vi "CRYReport Pic Get License.vi"() -> (0 "363d8b37-68c8-11db-be1e-0013d350667c":string, 2 "363d8b35-68c8-11db-be1e-0013d350667c":string)   [LabVIEW 2013]
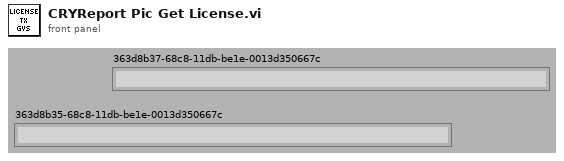
[diagram p1: front panel]
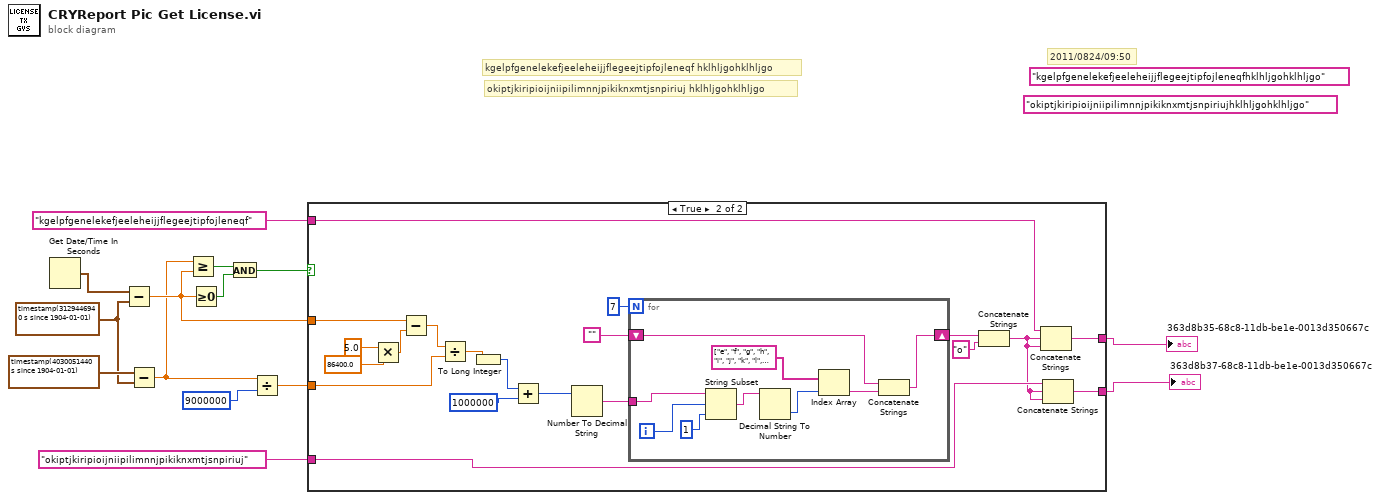
[diagram p0: block diagram]
diagram:
  w6 = timestamp(3129446940 s since 1904-01-01) ("current time")
  (unwired) "okiptjkiripioijniipilimnnjpikiknxmtjsnpiriujhklhljgohklhljgo"
  (unwired) "kgelpfgenelekefjeeleheijjflegeejtipfojleneqfhklhljgohklhljgo"
  # "2011/0824/09:50"
  # "okiptjkiripioijniipilimnnjpikiknxmtjsnpiriuj hklhljgohklhljgo"
  # "kgelpfgenelekefjeeleheijjflegeejtipfojleneqf hklhljgohklhljgo"
  n1 = Get Date/Time In Seconds() -> (seconds since 1Jan1904=w10:timestamp)
  n2 = Subtract(x=w10, y=w6) -> (x-y=w14:dbl)
  n3 = Subtract(x=timestamp(4030051440 s since 1904-01-01) ("current time"), y=w6) -> (x-y=w3:dbl)
  n4 = Greater Or Equal?(x=w3, y=w14) -> (x >= y?=w12:bool)
  n5 = Greater Or Equal To 0?(x=w14) -> (x >= 0?=w13:bool)
  n6 = And(x=w12, y=w13) -> (x .and. y?=w11:bool)
  n7 = Divide(x=w3, y=9000000) -> (x/y=w4:dbl)
  n8 = case shown="True" w11 {
    tunnel: w14 -> [_ w20]
    tunnel: [w16 w30] -> w2
    tunnel: "kgelpfgenelekefjeeleheijjflegeejtipfojleneqf" ("string") -> [w16 w29]
    tunnel: "okiptjkiripioijniipilimnnjpikiknxmtjsnpiriuj" ("string") -> [w15 w27]
    tunnel: [w15 w25] -> w1
    tunnel: w4 -> [_ w22]
    frame False {
    }
    frame True {
      n9 = Multiply(x=5.0, y=86400.0) -> (x*y=w19:dbl)
      n10 = Subtract(x=w20, y=w19) -> (x-y=w21:dbl)
      n11 = Divide(x=w21, y=w22) -> (x/y=w24:dbl)
      n12 = To Long Integer(number=w24) -> (32bit integer=w23:i32)
      n13 = Add(x=w23, y=1000000) -> (x+y=w28:i32)
      n14 = Number To Decimal String(number=w28) -> (decimal integer string=w35:string)  [unwired: 1 in]
      n15 = for {
        N: 7 -> [_]
        tunnel: w35 -> [w45]
        shift-right: [w38] -> w32
        shift-left: "" -> [w39]
        i -> [w43]
        n16 = String Subset(string=w45, offset (0)=w43, length (rest)=1 ("length (rest)")) -> (substring=w42:string)
        n17 = Decimal String To Number(string=w42) -> (number=w37:i32)  [unwired: 2 in, 1 out]
        n18 = Index Array(array=string[] ["e", "f", "g", "h", "i", "j", "k", "l", "m", "n"] ("Cannel Out"), index=w37) -> (element=w40:string)
        n19 = Concatenate Strings(w39, w40) -> (w38:string)
      }
      n20 = Concatenate Strings(w32, "o" ("string")) -> (w26:string)
      n21 = Concatenate Strings(w29, w26, w26) -> (w30:string)
      n22 = Concatenate Strings(w27, w26, w26) -> (w25:string)
    }
  }
  "363d8b35-68c8-11db-be1e-0013d350667c" <- w2
  "363d8b37-68c8-11db-be1e-0013d350667c" <- w1
